vi "SignalGen.vi"(4 "Output Waveform (Sine)":string(combo)="W1", 6 "Trigger Mode (Cont)":string(combo)="M1", 8 "Burst Count":dbl=50.0, 9 "Amplitide (V)":dbl=5.0, 10 "Modulation Frequency (Hz)":dbl, 11 "SG GPIB Address":i16=22) -> ()   [LabVIEW 2015]
doc: "VI preps the Wavetek Model 81 signal generators for use. Sets the operation frequency, amplitude, and set the unit for external burst triggering."
panel:
  out "error out":errorcluster
  in  "error in (no error)":errorcluster
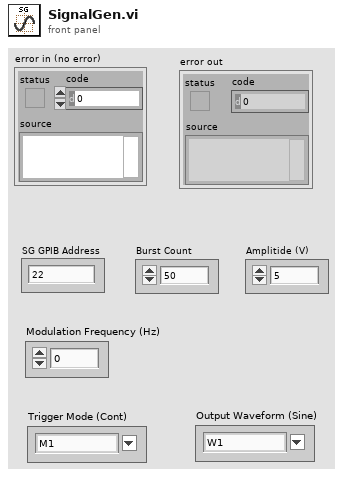
[diagram p1: front panel]
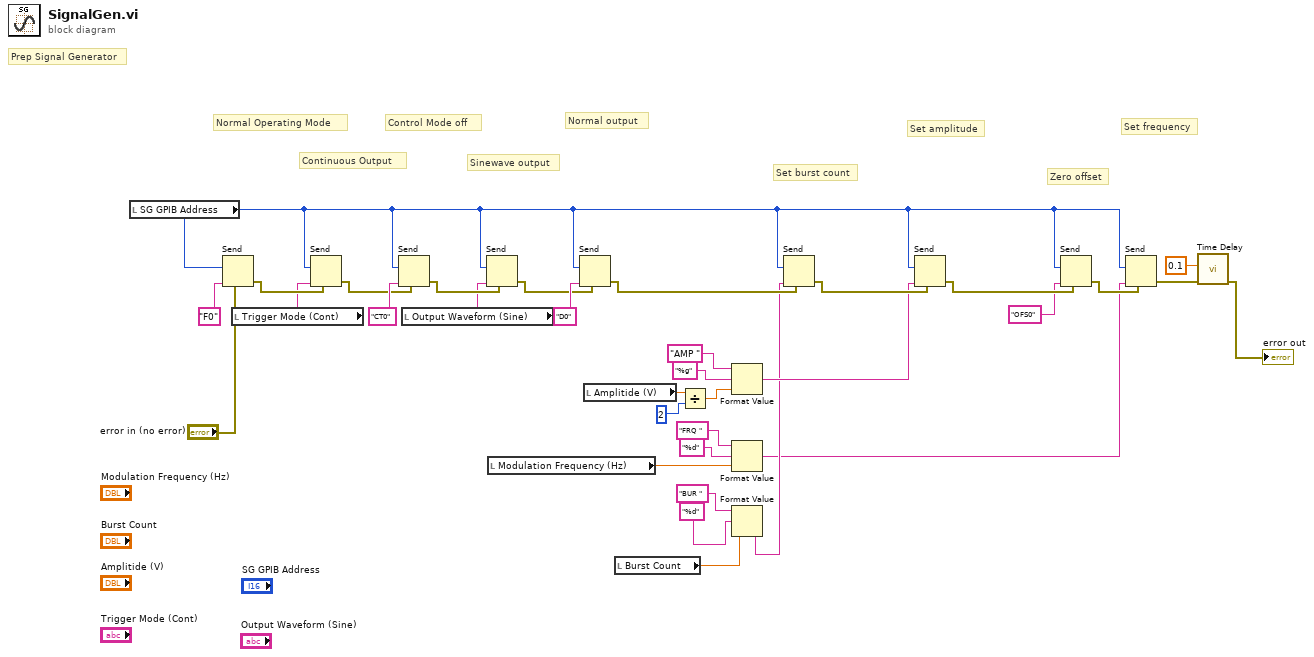
[diagram p0: block diagram]
diagram:
  # "Set frequency"
  # "Zero offset"
  # "Set amplitude"
  # "Set burst count"
  # "Normal output"
  # "Sinewave output"
  # "Control Mode off"
  # "Continuous Output"
  # "Normal Operating Mode"
  # "Prep Signal Generator"
  n1 = local read "SG GPIB Address"() -> (w5:i16)
  n2 = Send(2:w5, 4:"error in (no error)", 5:"F0") -> (8:w22:errorcluster)  [unwired: 2 in, 2 out]
  n3 = local read "Trigger Mode (Cont)"() -> (w2:string)
  n4 = Send(2:w5, 4:w22, 5:w2) -> (8:w21:errorcluster)  [unwired: 2 in, 2 out]
  n5 = Send(2:w5, 4:w21, 5:"CT0") -> (8:w20:errorcluster)  [unwired: 2 in, 2 out]
  n6 = local read "Output Waveform (Sine)"() -> (w1:string)
  n7 = Send(2:w5, 4:w20, 5:w1) -> (8:w19:errorcluster)  [unwired: 2 in, 2 out]
  n8 = local read "Modulation Frequency (Hz)"() -> (w24:dbl)
  n9 = Send(2:w5, 4:w19, 5:"D0") -> (8:w10:errorcluster)  [unwired: 2 in, 2 out]
  n10 = local read "Amplitide (V)"() -> (w30:dbl)
  n11 = local read "Burst Count"() -> (w11:dbl)
  n12 = Divide(x=w30, y=2) -> (x/y=w29:dbl)
  n13 = Format Value(string ("")="AMP ", format string="%g", value (0)=w29) -> (output string=w9:string)
  n14 = Format Value(string ("")="FRQ ", format string="%d", value (0)=w24) -> (output string=w6:string)
  n15 = Format Value(string ("")="BUR ", format string="%d", value (0)=w11) -> (output string=w7:string)
  n16 = Send(2:w5, 4:w10, 5:w7) -> (8:w18:errorcluster)  [unwired: 2 in, 2 out]
  n17 = Send(2:w5, 4:w18, 5:w9) -> (8:w17:errorcluster)  [unwired: 2 in, 2 out]
  n18 = Send(2:w5, 4:w17, 5:"OFS0") -> (8:w14:errorcluster)  [unwired: 2 in, 2 out]
  n19 = Send(2:w5, 4:w14, 5:w6) -> (8:w12:errorcluster)  [unwired: 2 in, 2 out]
  n20 = call "Time Delay"("error in (no error)"=w12, "Delay Time (s)"=0.1) -> ("error out"=→"error out":errorcluster)  [unwired: 9 in]
